vi "Init Base.vi"(8 "Error In":errorcluster, 11 "object in":refnum<class "Instrument.lvclass">) -> (0 "Error Out":errorcluster, 3 "object out":refnum<class "Instrument.lvclass">)   [LabVIEW 2023, in "HAL.lvlib" / "Instrument.lvclass"]
uses:
  Instrument.lvclass
  Instrument.lvclass/Instrument.ctl
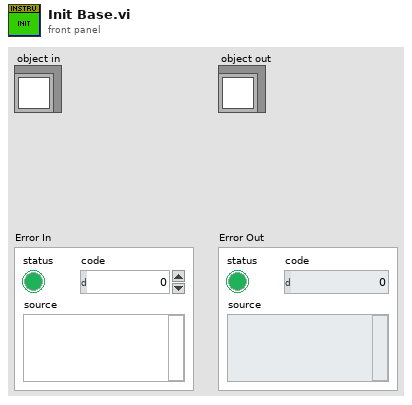
[diagram p1: front panel]
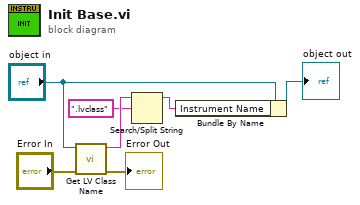
[diagram p0: block diagram]
diagram:
  n1 = call <vilib>:"Get LV Class Name.vi"("error in (no error)"="Error In", "object"="object in") -> ("error out"=→"Error Out":errorcluster, "class name"=w6:string)  [unwired: 8 in]
  n2 = Search/Split String(string=w6, search string/char (-)=".lvclass") -> (substring before match=w2:string)  [unwired: 1 in, 2 out]
  n3 = Bundle By Name(cluster="object in", "Instrument Name"=w2) -> (→"object out":refnum<class "Instrument.lvclass">)
